vi "Write Section Cluster.vi"(6 "Section Name (Cluster Name)":string, 7 "error in (no error)":errorcluster, 8 "Section Cluster":variant, 10 "JSON Sections":string="{}") -> (0 "error out":errorcluster, 3 "<JSON>":string caption="<JSON>Sections")   [LabVIEW 2020, in "JSONtext.lvlib"]
doc: "Merges a Section Cluster into JSON Object. A \"Section Cluster\" is defined in analogy to the OpenG Variant Config Library \"Section Cluster\" functions, using a JSON Object, with subObjects representing \"Sections\", instead of INI format.\n\nMerging means that each element of the Section Cluster is inserted into the JSON \"Section\" (Object Item), using the data name of the cluster element. If a Path to the Section is not specified then the data name of the cluster is used. The Section is created if it does not exist.\n\nFor example, Merging the Cluster \"Settings\" with elements A=123 and B=\"test\" into {\"C\":2,\"Settings\":{\"A\"=6,\"D\":9}} would result in:\n{\"C\":2,\"Settings\":{\"A\"=123,\"D\":9,\"B\":\"test\"}}\n\nNote that this merging is not recursive into subClusters."
uses:
  <vilib>/JDP Science/JSONtext/JSONtext.lvlib
  <vilib>/Utility/Data Type/NI_Data Type.lvlib
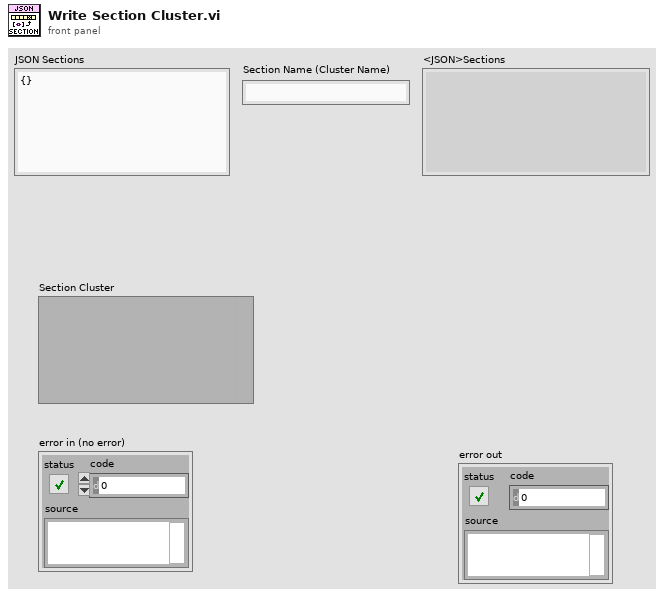
[diagram p1: front panel]
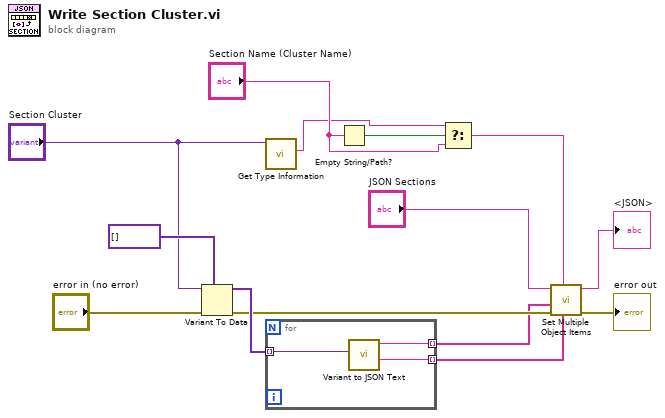
[diagram p0: block diagram]
diagram:
  n1 = Variant To Data(error in="error in (no error)", type=variant[] [], Variant="Section Cluster") -> (data=w10:variant[], error out=w8:errorcluster)
  n2 = call <vilib>:"Get Type Information.vi"("variant"="Section Cluster") -> ("name"=w1:string)  [unwired: 6 in, 4 out]
  n3 = for {
    tunnel: w10 -> [w17] mode=indexing
    tunnel: [w16] -> w6 mode=indexing
    tunnel: [w15] -> w7 mode=indexing
    n4 = call <vilib>:"Variant to JSON Text.vi"("Variant"=w17) -> ("Name of data in Variant"=w16:string, "<JSON>"=w15:string)  [unwired: 8 in, 1 out]
  }
  n5 = Empty String/Path?(string/path="Section Name (Cluster Name)") -> (empty?=w4:bool)
  n6 = Select(t=w1, s=w4, f="Section Name (Cluster Name)") -> (s? t:f=w3:string)
  n7 = call <vilib>:"Set Multiple Object Items.vi"("Item Names"=w6, "$Path or Item Name"=w3, "error in (no error)"=w8, "JSON Items"=w7, "JSON"="JSON Sections") -> ("error out"=→"error out":errorcluster, "<JSON>"=→"<JSON>":string)  [unwired: 4 in]
